vi "Add Label.vi"(8 "error in":errorcluster, 10 "label configuration":T1 {"sdi" items=["All", "Item00", "Item01", "Item10", "Item11"]}, 11 "channel in":refnum<k24>) -> (0 "error out":errorcluster, 2 "new label":refnum<k24>, 3 "channel out":refnum<k24>)   [LabVIEW 2020, in "AIM_429_Parameter_ni.lvlib"]
uses:
  AIM_429_Parameter_ni.lvlib
  C:/Users/Administrator/Desktop/GIT/Ballard-Arinc-429-XML-Generator/Source/Assemblies/Aim_429_Parameter_ni/bin/Debug/AIM_429_Parameter_ni.dll
  Assemblies/Aim_429_Parameter_ni/bin/Debug/AIM_429_Parameter_ni.dll
  _tyedefs/label_type.ctl
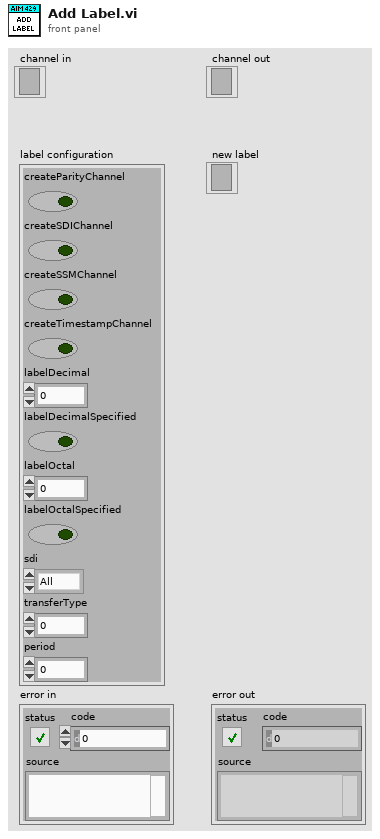
[diagram p1: front panel]
types:
  T1 = typedef "AIM_429_Parameter_ni.lvlib/label_type.ctl" = cluster{"createParityChannel":bool, "createSDIChannel":bool, "createSSMChannel":bool, "createTimestampChannel":bool, "labelDecimal":i32, "labelDecimalSpecified":bool, "labelOctal":i32, "labelOctalSpecified":bool, "sdi":i32, "transferType":i32, "period":i32}
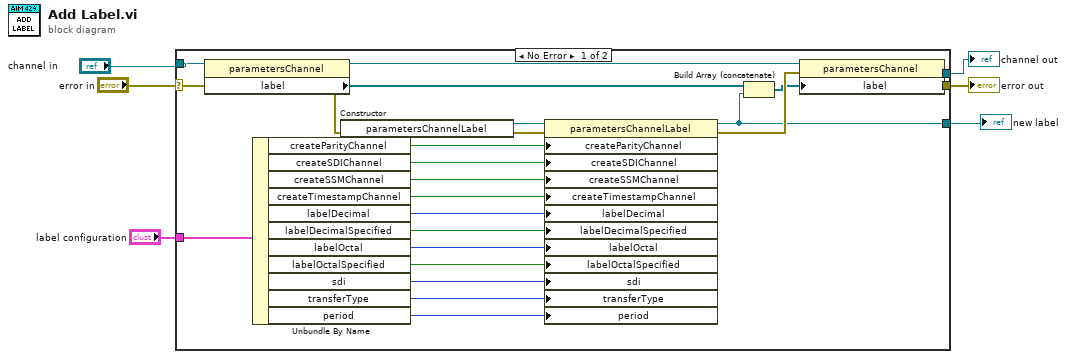
[diagram p0: block diagram]
diagram:
  n1 = case shown="No Error" "error in" {
    selector: "error in" -> [w29 w31]
    tunnel: [w25 w32] -> w6
    tunnel: [w24 w31] -> w5
    tunnel: "channel in" -> [w30 w32]
    tunnel: [w9 _] -> w1
    tunnel: "label configuration" -> [w20 _]
    frame No Error {
      n2 = property class="parametersChannel"(reference=w30, error in=w29) -> (reference out=w26:refnum<k24>, error out=w27:errorcluster, "label"=w28:refnum<k24>[])
      n3 = Unbundle By Name(w20) -> ("createParityChannel"=w19:bool, "createSDIChannel"=w18:bool, "createSSMChannel"=w17:bool, "createTimestampChannel"=w16:bool, "labelDecimal"=w15:i32, "labelDecimalSpecified"=w14:bool, "labelOctal"=w13:i32, "labelOctalSpecified"=w12:bool, "sdi"=w11:i32, "transferType"=w10:i32, "period"=w7:i32)
      n4 = constructor class="parametersChannelLabel"(error in=w27) -> (reference out=w23:refnum<k24>, error out=w22:errorcluster)  [unwired: 2 in, 1 out]
      n5 = property class="parametersChannelLabel"(reference=w23, error in=w22, "createParityChannel"=w19, "createSDIChannel"=w18, "createSSMChannel"=w17, "createTimestampChannel"=w16, "labelDecimal"=w15, "labelDecimalSpecified"=w14, "labelOctal"=w13, "labelOctalSpecified"=w12, "sdi"=w11, "transferType"=w10, "period"=w7) -> (reference out=w9:refnum<k24>, error out=w21:errorcluster)
      n6 = Build Array (concatenate)(w28, w9) -> (w8:refnum<k24>[])
      n7 = property class="parametersChannel"(reference=w26, error in=w21, "label"=w8) -> (reference out=w25:refnum<k24>, error out=w24:errorcluster)
    }
    frame Error {
    }
  }
  "channel out" <- w6
  "error out" <- w5
  "new label" <- w1
